vi "SSC Digital Write Sequencer Register.vi"(0 "Digital SSC in":T1[](array[typedef]), 5 "Sequencer Register":string(combo)="reg0", 7 "Value (0)":i32, 11 "error in":errorcluster) -> (4 "Digital SSC out":T1[](array[typedef]), 15 "error out":errorcluster)   [LabVIEW 2020]
doc: "Writes a value to a pattern sequencer register on the device(s) connected to the specified pin(s) and pin group(s). Use pattern sequencer registers to pass numeric values between the pattern sequencer and a runtime test program."
uses:
  SSC Digital.ctl
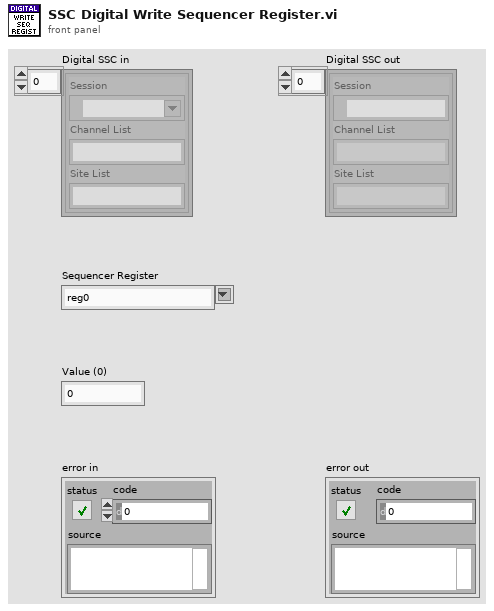
[diagram p1: front panel]
types:
  T1 = typedef "SSC Digital.ctl" = cluster{"Session":refnum<k15>, "Channel List":string, "Site List":string}
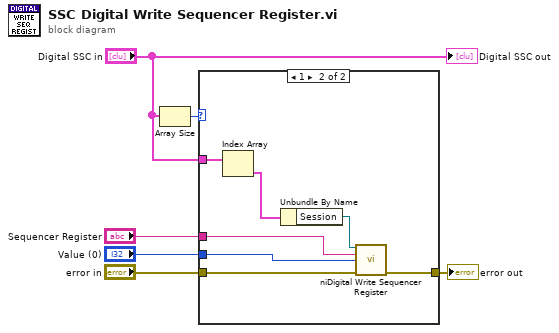
[diagram p0: block diagram]
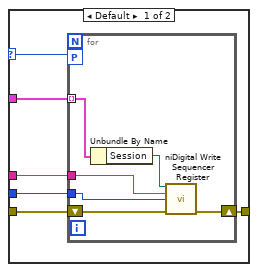
[diagram p2: hidden frame]
diagram:
  n1 = Array Size(array="Digital SSC in") -> (size(s)=w2:i32)
  n2 = case shown="1" w2 {
    selector: w2 -> [w8 _]
    tunnel: "error in" -> [w12 w25]
    tunnel: "Value (0)" -> [w11 w24]
    tunnel: "Sequencer Register" -> [w10 w23]
    tunnel: [w9 w22] -> w3
    tunnel: "Digital SSC in" -> [w7 w21]
    frame Default {
      n3 = for {
        tunnel: w11 -> [w16]
        workers-P: w8 -> [_]
        tunnel: w10 -> [w15]
        shift-right: [w17] -> w9
        shift-left: w12 -> [w18]
        tunnel: w7 -> [w14] mode=indexing
        n4 = Unbundle By Name(w14) -> ("Session"=w13:refnum<k15>)
        n5 = call <instrlib>:"niDigital Write Sequencer Register.vi"("instrument handle"=w13, "sequencer register"=w15, "value"=w16, "error in"=w18) -> ("error out"=w17:errorcluster)  [unwired: 10 in, 1 out]
      }
    }
    frame 1 {
      n6 = Index Array(array=w21) -> (element=w19:T1)  [unwired: 1 in]
      n7 = Unbundle By Name(w19) -> ("Session"=w20:refnum<k15>)
      n8 = call <instrlib>:"niDigital Write Sequencer Register.vi"("instrument handle"=w20, "sequencer register"=w23, "value"=w24, "error in"=w25) -> ("error out"=w22:errorcluster)  [unwired: 10 in, 1 out]
    }
  }
  "error out" <- w3
  "Digital SSC out" <- "Digital SSC in"
